vi "canDataSort.vi"() -> ()   [LabVIEW 2023] (continued)
      30\t75\tE0\t2E\t80\tFF\tFF\tFD\r\n      4322  0CF101A7   00000004    8        68\t00\t97\tCC\t00\t19\t39\tF2\r\n      4322  1FFFFFFF   00000004    8        00\t00\tFF\tFF\tFF\tFF\tFF\tFF\r\n      4312  1FFFFFFF   00000004    8        00\t20\tFF\tFF\tFF\tFF\tFF\tFF\r\n      4303  0CF102A7   00000004    8        30\t75\tE0\t2E\t80\tFF\tFF\tFD\r\n      4303  0CF101A7   00000004    8        68\t00\t97\tCC\t00\t19\t39\tF1\r\n      4302  1FFFFFFF   00000004    8        00\t00\tFF\tFF\tFF\tFF\tFF\tFF\r\n      4343  0C3C4D4A   00000004    8        BE\tFF\tFF\t7F\t18\tFF\tFF\t63\r\n      4343  0CF101A7   00000004    8        68\t00\t97\tCC\t00\t19\t39\tF3\r\n      4342  18F120F0   00000004    8        2B\t75\t60\tB1\tB0\t01\tFF\tFF\r\n      4341  18F11FF0   00000004    8        FF\t3F\t90\t68\t88\t1B\t10\t3C\r\n      4332  1FFFFFFF   00000004    8        00\t20\tFF\tFF\tFF\tFF\tFF\tFF\r\n      4323  0CF102A7   00000004    8        30\t75\tE0\t2E\t80\tFF\tFF\tFD\r\n      4322  0CF101A7   00000004    8        68\t00\t97\tCC\t00\t19\t39\tF2\r\n      4322  1FFFFFFF   00000004    8        00\t00\tFF\tFF\tFF\tFF\tFF\tFF\r\n      4312  1FFFFFFF   00000004    8        00\t20\tFF\tFF\tFF\tFF\tFF\tFF\r\n      4303  0CF102A7   00000004    8        30\t75\tE0\t2E\t80\tFF\tFF\tFD\r\n      4303  0CF101A7   00000004    8        68\t00\t97\tCC\t00\t19\t39\tF1\r\n      4344  0CF102A7   00000004    8        30\t75\tE0\t2E\t80\tFF\tFF\tFD\r\n      4343  0C3C4D4A   00000004    8        BE\tFF\tFF\t7F\t18\tFF\tFF\t63\r\n      4343  0CF101A7   00000004    8        68\t00\t97\tCC\t00\t19\t39\tF3\r\n      4342  18F120F0   00000004    8        2B\t75\t60\tB1\tB0\t01\tFF\tFF\r\n      4341  18F11FF0   00000004    8        FF\t3F\t90\t68\t88\t1B\t10\t3C\r\n      4332  1FFFFFFF   00000004    8        00\t20\tFF\tFF\tFF\tFF\tFF\tFF\r\n      4323  0CF102A7   00000004    8        30\t75\tE0\t2E\t80\tFF\tFF\tFD\r\n      4322  0CF101A7   00000004    8        68\t00\t97\tCC\t00\t19\t39\tF2\r\n      4322  1FFFFFFF   00000004    8        00\t00\tFF\tFF\tFF\tFF\tFF\tFF\r\n      4312  1FFFFFFF   00000004    8        00\t20\tFF\tFF\tFF\tFF\tFF\tFF\r\n      4303  0CF102A7   00000004    8        30\t75\tE0\t2E\t80\tFF\tFF\tFD\r\n      4344  0CF103A7   00000004    8        17\t1F\t08\t60\tB1\t1F\t08\t63\r\n      4344  0CF102A7   00000004    8        30\t75\tE0\t2E\t80\tFF\tFF\tFD\r\n      4343  0C3C4D4A   00000004    8        BE\tFF\tFF\t7F\t18\tFF\tFF\t63\r\n      4343  0CF101A7   00000004    8        68\t00\t97\tCC\t00\t19\t39\tF3\r\n      4342  18F120F0   00000004    8        2B\t75\t60\tB1\tB0\t01\tFF\tFF\r\n      4341  18F11FF0   00000004    8        FF\t3F\t90\t68\t88\t1B\t10\t3C\r\n      4332  1FFFFFFF   00000004    8        00\t20\tFF\tFF\tFF\tFF\tFF\tFF\r\n      4323  0CF102A7   00000004    8        30\t75\tE0\t2E\t80\tFF\tFF\tFD\r\n      4322  0CF101A7   00000004    8        68\t00\t97\tCC\t00\t19\t39\tF2\r\n      4322  1FFFFFFF   00000004    8        00\t00\tFF\tFF\tFF\tFF\tFF\tFF\r\n      4312  1FFFFFFF   00000004    8        00\t20\tFF\tFF\tFF\tFF\tFF\tFF\r\n      4345  0CF104A7   00000004    8        F0\t60\t22\tFC\tFF\tFF\tFF\t63\r\n      4344  0CF103A7   00000004    8        17\t1F\t08\t60\tB1\t1F\t08\t63\r\n      4344  0CF102A7   00000004    8        30\t75\tE0\t2E\t80\tFF\tFF\tFD\r\n      4343  0C3C4D4A   00000004    8        BE\tFF\tFF\t7F\t18\tFF\tFF\t63\r\n      4343  0CF101A7   00000004    8        68\t00\t97\tCC\t00\t19\t39\tF3\r\n      4342  18F120F0   00000004    8        2B\t75\t60\tB1\tB0\t01\tFF\tFF\r\n      4341  18F11FF0   00000004    8        FF\t3F\t90\t68\t88\t1B\t10\t3C\r\n      4332  1FFFFFFF   00000004    8        00\t20\tFF\tFF\tFF\tFF\tFF\tFF\r\n      4323  0CF102A7   00000004    8        30\t75\tE0\t2E\t80\tFF\tFF\tFD\r\n      4322  0CF101A7   00000004    8        68\t00\t97\tCC\t00\t19\t39\tF2\r\n      4322  1FFFFFFF   00000004    8        00\t00\tFF\tFF\tFF\tFF\tFF\tFF\r\n      4345  18F106A7   00000004    8        00\tF7\tFF\tFF\tFF\tFF\tFF\tC7\r\n      4345  0CF104A7   00000004    8        F0\t60\t22\tFC\tFF\tFF\tFF\t63\r\n      4344  0CF103A7   00000004    8        17\t1F\t08\t60\tB1\t1F\t08\t63\r\n      4344  0CF102A7   00000004    8        30\t75\tE0\t2E\t80\tFF\tFF\tFD\r\n      4343  0C3C4D4A   00000004    8        BE\tFF\tFF\t7F\t18\tFF\tFF\t63\r\n      4343  0CF101A7   00000004    8        68\t00\t97\tCC\t00\t19\t39\tF3\r\n      4342  18F120F0   00000004    8        2B\t75\t60\tB1\tB0\t01\tFF\tFF\r\n      4341  18F11FF0   00000004    8        FF\t3F\t90\t68\t88\t1B\t10\t3C\r\n      4332  1FFFFFFF   00000004    8        00\t20\tFF\tFF\tFF\tFF\tFF\tFF\r\n      4323  0CF102A7   00000004    8        30\t75\tE0\t2E\t80\tFF\tFF\tFD\r\n      4322  0CF101A7   00000004    8        68\t00\t97\tCC\t00\t19\t39\tF2\r\n      4346  18F121F0   00000004    8        09\t34\t00\t00\tFF\tFF\tB0\t01\r\n      4345  18F106A7   00000004    8        00\tF7\tFF\tFF\tFF\tFF\tFF\tC7\r\n      4345  0CF104A7   00000004    8        F0\t60\t22\tFC\tFF\tFF\tFF\t63\r\n      4344  0CF103A7   00000004    8        17\t1F\t08\t60\tB1\t1F\t08\t63\r\n      4344  0CF102A7   00000004    8        30\t75\tE0\t2E\t80\tFF\tFF\tFD\r\n      4343  0C3C4D4A   00000004    8        BE\tFF\tFF\t7F\t18\tFF\tFF\t63\r\n      4343  0CF101A7   00000004    8        68\t00\t97\tCC\t00\t19\t39\tF3\r\n      4342  18F120F0   00000004    8        2B\t75\t60\tB1\tB0\t01\tFF\tFF\r\n      4341  18F11FF0   00000004    8        FF\t3F\t90\t68\t88\t1B\t10\t3C\r\n      4332  1FFFFFFF   00000004    8        00\t20\tFF\tFF\tFF\tFF\tFF\tFF\r\n      4323  0CF102A7   00000004    8        30\t75\tE0\t2E\t80\tFF\tFF\tFD\r\n      4346  1FFFFFFF   00000004    8        00\t20\tFF\tFF\tFF\tFF\tFF\tFF\r\n      4346  18F121F0   00000004    8        09\t34\t00\t00\tFF\tFF\tB0\t01\r\n      4345  18F106A7   00000004    8        00\tF7\tFF\tFF\tFF\tFF\tFF\tC7\r\n      4345  0CF104A7   00000004    8        F0\t60\t22\tFC\tFF\tFF\tFF\t63\r\n      4344  0CF103A7   00000004    8        17\t1F\t08\t60\tB1\t1F\t08\t63\r\n      4344  0CF102A7   00000004    8        30\t75\tE0\t2E\t80\tFF\tFF\tFD\r\n      4343  0C3C4D4A   00000004    8        BE\tFF\tFF\t7F\t18\tFF\tFF\t63\r\n      4343  0CF101A7   00000004    8        68\t00\t97\tCC\t00\t19\t39\tF3\r\n      4342  18F120F0   00000004    8        2B\t75\t60\tB1\tB0\t01\tFF\tFF\r\n      4341  18F11FF0   00000004    8        FF\t3F\t90\t68\t88\t1B\t10\t3C\r\n      4332  1FFFFFFF   00000004    8        00\t20\tFF\tFF\tFF\tFF\tFF\tFF\r\n      4352  1FFFFFFF   00000004    8        00\t00\tFF\tFF\tFF\tFF\tFF\tFF\r\n      4346  1FFFFFFF   00000004    8        00\t20\tFF\tFF\tFF\tFF\tFF\tFF\r\n      4346  18F121F0   00000004    8        09\t34\t00\t00\tFF\tFF\tB0\t01\r\n      4345  18F106A7   00000004    8        00\tF7\tFF\tFF\tFF\tFF\tFF\tC7\r\n      4345  0CF104A7   00000004    8        F0\t60\t22\tFC\tFF\tFF\tFF\t63\r\n      4344  0CF103A7   00000004    8        17\t1F\t08\t60\tB1\t1F\t08\t63\r\n      4344  0CF102A7   00000004    8        30\t75\tE0\t2E\t80\tFF\tFF\tFD\r\n      4343  0C3C4D4A   00000004    8        BE\tFF\tFF\t7F\t18\tFF\tFF\t63\r\n      4343  0CF101A7   00000004    8        68\t00\t97\tCC\t00\t19\t39\tF3\r\n      4342  18F120F0   00000004    8        2B\t75\t60\tB1\tB0\t01\tFF\tFF\r\n      4341  18F11FF0   00000004    8        FF\t3F\t90\t68\t88\t1B\t10\t3C\r\n      4362  1FFFFFFF   00000004    8        00\t00\tFF\tFF\tFF\tFF\tFF\tFF\r\n      4352  1FFFFFFF   00000004    8        00\t00\tFF\tFF\tFF\tFF\tFF\tFF\r\n      4346  1FFFFFFF   00000004    8        00\t20\tFF\tFF\tFF\tFF\tFF\tFF\r\n      4346  18F121F0   00000004    8        09\t34\t00\t00\tFF\tFF\tB0\t01\r\n      4345  18F106A7   00000004    8        00\tF7\tFF\tFF\tFF\tFF\tFF\tC7\r\n      4345  0CF104A7   00000004    8        F0\t60\t22\tFC\tFF\tFF\tFF\t63\r\n      4344  0CF103A7   00000004    8        17\t1F\t08\t60\tB1\t1F\t08\t63\r\n      4344  0CF102A7   00000004    8        30\t75\tE0\t2E\t80\tFF\tFF\tFD\r\n      4343  0C3C4D4A   00000004    8        BE\tFF\tFF\t7F\t18\tFF\tFF\t63\r\n      4343  0CF101A7   00000004    8        68\t00\t97\tCC\t00\t19\t39\tF3\r\n      4342  18F120F0   00000004    8        2B\t75\t60\tB1\tB0\t01\tFF\tFF\r\n      4363  0CF101A7   00000004    8        68\t00\t97\tCC\t00\t19\t39\tF4\r\n      4362  1FFFFFFF   00000004    8        00\t00\tFF\tFF\tFF\tFF\tFF\tFF\r\n      4352  1FFFFFFF   00000004    8        00\t00\tFF\tFF\tFF\tFF\tFF\tFF\r\n      4346  1FFFFFFF   00000004    8        00\t20\tFF\tFF\tFF\tFF\tFF\tFF\r\n      4346  18F121F0   00000004    8        09\t34\t00\t00\tFF\tFF\tB0\t01\r\n      4345  18F106A7   00000004    8        00\tF7\tFF\tFF\tFF\tFF\tFF\tC7\r\n      4345  0CF104A7   00000004    8        F0\t60\t22\tFC\tFF\tFF\tFF\t63\r\n      4344  0CF103A7   00000004    8        17\t1F\t08\t60\tB1\t1F\t08\t63\r\n      4344  0CF102A7   00000004    8        30\t75\tE0\t2E\t80\tFF\tFF\tFD\r\n      4343  0C3C4D4A   00000004    8        BE\tFF\tFF\t7F\t18\tFF\tFF\t63\r\n      4343  0CF101A7   00000004    8        68\t00\t97\tCC\t00\t19\t39\tF3\r\n      4363  0CF102A7   00000004    8        30\t75\tE0\t2E\t80\tFF\tFF\tFD\r\n      4363  0CF101A7   00000004    8        68\t00\t97\tCC\t00\t19\t39\tF4\r\n      4362  1FFFFFFF   00000004    8        00\t00\tFF\tFF\tFF\tFF\tFF\tFF\r\n      4352  1FFFFFFF   00000004    8        00\t00\tFF\tFF\tFF\tFF\tFF\tFF\r\n      4346  1FFFFFFF   00000004    8        00\t20\tFF\tFF\tFF\tFF\tFF\tFF\r\n      4346  18F121F0   00000004    8        09\t34\t00\t00\tFF\tFF\tB0\t01\r\n      4345  18F106A7   00000004    8        00\tF7\tFF\tFF\tFF\tFF\tFF\tC7\r\n      4345  0CF104A7   00000004    8        F0\t60\t22\tFC\tFF\tFF\tFF\t63\r\n      4344  0CF103A7   00000004    8        17\t1F\t08\t60\tB1\t1F\t08\t63\r\n      4344  0CF102A7   00000004    8        30\t75\tE0\t2E\t80\tFF\tFF\tFD\r\n      4343  0C3C4D4A   00000004    8        BE\tFF\tFF\t7F\t18\tFF\tFF\t63\r\n      4372  1FFFFFFF   00000004    8        00\t00\tFF\tFF\tFF\tFF\tFF\tFF\r\n      4363  0CF102A7   00000004    8        30\t75\tE0\t2E\t80\tFF\tFF\tFD\r\n      4363  0CF101A7   00000004    8        68\t00\t97\tCC\t00\t19\t39\tF4\r\n      4362  1FFFFFFF   00000004    8        00\t00\tFF\tFF\tFF\tFF\tFF\tFF\r\n      4352  1FFFFFFF   00000004    8        00\t00\tFF\tFF\tFF\tFF\tFF\tFF\r\n      4346  1FFFFFFF   00000004    8        00\t20\tFF\tFF\tFF\tFF\tFF\tFF\r\n      4346  18F121F0   00000004    8        09\t34\t00\t00\tFF\tFF\tB0\t01\r\n      4345  18F106A7   00000004    8        00\tF7\tFF\tFF\tFF\tFF\tFF\tC7\r\n      4345  0CF104A7   00000004    8        F0\t60\t22\tFC\tFF\tFF\tFF\t63\r\n      4344  0CF103A7   00000004    8        17\t1F\t08\t60\tB1\t1F\t08\t63\r\n      4344  0CF102A7   00000004    8        30\t75\tE0\t2E\t80\tFF\tFF\tFD\r\n      4382  1FFFFFFF   00000004    8        00\t00\tFF\tFF\tFF\tFF\tFF\tFF\r\n      4372  1FFFFFFF   00000004    8        00\t00\tFF\tFF\tFF\tFF\tFF\tFF\r\n      4363  0CF102A7   00000004    8        30\t75\tE0\t2E\t80\tFF\tFF\tFD\r\n      4363  0CF101A7   00000004    8        68\t00\t97\tCC\t00\t19\t39\tF4\r\n      4362  1FFFFFFF   00000004    8        00\t00\tFF\tFF\tFF\tFF\tFF\tFF\r\n      4352  1FFFFFFF   00000004    8        00\t00\tFF\tFF\tFF\tFF\tFF\tFF\r\n      4346  1FFFFFFF   00000004    8        00\t20\tFF\tFF\tFF\tFF\tFF\tFF\r\n      4346  18F121F0   00000004    8        09\t34\t00\t00\tFF\tFF\tB0\t01\r\n      4345  18F106A7   00000004    8        00\tF7\tFF\tFF\tFF\tFF\tFF\tC7\r\n      4345  0CF104A7   00000004    8        F0\t60\t22\tFC\tFF\tFF\tFF\t63\r\n      4344  0CF103A7   00000004    8        17\t1F\t08\t60\tB1\t1F\t08\t63\r\n      4382  0CF101A7   00000004    8        68\t00\t97\tCC\t00\t19\t39\tF5\r\n      4382  1FFFFFFF   00000004    8        00\t00\tFF\tFF\tFF\tFF\tFF\tFF\r\n      4372  1FFFFFFF   00000004    8        00\t00\tFF\tFF\tFF\tFF\tFF\tFF\r\n      4363  0CF102A7   00000004    8        30\t75\tE0\t2E\t80\tFF\tFF\tFD\r\n      4363  0CF101A7   00000004    8        68\t00\t97\tCC\t00\t19\t39\tF4\r\n      4362  1FFFFFFF   00000004    8        00\t00\tFF\tFF\tFF\tFF\tFF\tFF\r\n      4352  1FFFFFFF   00000004    8        00\t00\tFF\tFF\tFF\tFF\tFF\tFF\r\n      4346  1FFFFFFF   00000004    8        00\t20\tFF\tFF\tFF\tFF\tFF\tFF\r\n      4346  18F121F0   00000004    8        09\t34\t00\t00\tFF\tFF\tB0\t01\r\n      4345  18F106A7   00000004    8        00\tF7\tFF\tFF\tFF\tFF\tFF\tC7\r\n      4345  0CF104A7   00000004    8        F0\t60\t22\tFC\tFF\tFF\tFF\t63\r\n      4383  0CF102A7   00000004    8        30\t75\tE0\t2E\t80\tFF\tFF\tFD\r\n      4382  0CF101A7   00000004    8        68\t00\t97\tCC\t00\t19\t39\tF5\r\n      4382  1FFFFFFF   00000004    8        00\t00\tFF\tFF\tFF\tFF\tFF\tFF\r\n      4372  1FFFFFFF   00000004    8        00\t00\tFF\tFF\tFF\tFF\tFF\tFF\r\n      4363  0CF102A7   00000004    8        30\t75\tE0\t2E\t80\tFF\tFF\tFD\r\n      4363  0CF101A7   00000004    8        68\t00\t97\tCC\t00\t19\t39\tF4\r\n      4362  1FFFFFFF   00000004    8        00\t00\tFF\tFF\tFF\tFF\tFF\tFF\r\n      4352  1FFFFFFF   00000004    8        00\t00\tFF\tFF\tFF\tFF\tFF\tFF\r\n      4346  1FFFFFFF   00000004    8        00\t20\tFF\tFF\tFF\tFF\tFF\tFF\r\n      4346  18F121F0   00000004    8        09\t34\t00\t00\tFF\tFF\tB0\t01\r\n      4345  18F106A7   00000004    8        00\tF7\tFF\tFF\tFF\tFF\tFF\tC7\r\n      4392  1FFFFFFF   00000004    8        00\t00\tFF\tFF\tFF\tFF\tFF\tFF\r\n      4383  0CF102A7   00000004    8        30\t75\tE0\t2E\t80\tFF\tFF\tFD\r\n      4382  0CF101A7   00000004    8        68\t00\t97\tCC\t00\t19\t39\tF5\r\n      4382  1FFFFFFF   00000004    8        00\t00\tFF\tFF\tFF\tFF\tFF\tFF\r\n      4372  1FFFFFFF   00000004    8        00\t00\tFF\tFF\tFF\tFF\tFF\tFF\r\n      4363  0CF102A7   00000004    8        30\t75\tE0\t2E\t80\tFF\tFF\tFD\r\n      4363  0CF101A7   00000004    8        68\t00\t97\tCC\t00\t19\t39\tF4\r\n      4362  1FFFFFFF   00000004    8        00\t00\tFF\tFF\tFF\tFF\tFF\tFF\r\n      4352  1FFFFFFF   00000004    8        00\t00\tFF\tFF\tFF\tFF\tFF\tFF\r\n      4346  1FFFFFFF   00000004    8        00\t20\tFF\tFF\tFF\tFF\tFF\tFF\r\n      4346  18F121F0   00000004    8        09\t34\t00\t00\tFF\tFF\tB0\t01\r\n      4393  18F106A7   00000004    8        00\tF7\tFF\tFF\tFF\tFF\tFF\tC8\r\n      4392  1FFFFFFF   00000004    8        00\t00\tFF\tFF\tFF\tFF\tFF\tFF\r\n      4383  0CF102A7   00000004    8        30\t75\tE0\t2E\t80\tFF\tFF\tFD\r\n      4382  0CF101A7   00000004    8        68\t00\t97\tCC\t00\t19\t39\tF5\r\n      4382  1FFFFFFF   00000004    8        00\t00\tFF\tFF\tFF\tFF\tFF\tFF\r\n      4372  1FFFFFFF   00000004    8        00\t00\tFF\tFF\tFF\tFF\tFF\tFF\r\n      4363  0CF102A7   00000004    8        30\t75\tE0\t2E\t80\tFF\tFF\tFD\r\n      4363  0CF101A7   00000004    8        68\t00\t97\tCC\t00\t19\t39\tF4\r\n      4362  1FFFFFFF   00000004    8        00\t00\tFF\tFF\tFF\tFF\tFF\tFF\r\n      4352  1FFFFFFF   00000004    8        00\t00\tFF\tFF\tFF\tFF\tFF\tFF\r\n      4346  1FFFFFFF   00000004    8        00\t20\tFF\tFF\tFF\tFF\tFF\tFF\r\n      4402  1FFFFFFF   00000004    8        00\t00\tFF\tFF\tFF\tFF\tFF\tFF\r\n      4393  18F106A7   00000004    8        00\tF7\tFF\tFF\tFF\tFF\tFF\tC8\r\n      4392  1FFFFFFF   00000004    8        00\t00\tFF\tFF\tFF\tFF\tFF\tFF\r\n      4383  0CF102A7   00000004    8        30\t75\tE0\t2E\t80\tFF\tFF\tFD\r\n      4382  0CF101A7   00000004    8        68\t00\t97\tCC\t00\t19\t39\tF5\r\n      4382  1FFFFFFF   00000004    8        00\t00\tFF\tFF\tFF\tFF\tFF\tFF\r\n      4372  1FFFFFFF   00000004    8        00\t00\tFF\tFF\tFF\tFF\tFF\tFF\r\n      4363  0CF102A7   00000004    8        30\t75\tE0\t2E\t80\tFF\tFF\tFD\r\n      4363  0CF101A7   00000004    8        68\t00\t97\tCC\t00\t19\t39\tF4\r\n      4362  1FFFFFFF   00000004    8        00\t00\tFF\tFF\tFF\tFF\tFF\tFF\r\n      4352  1FFFFFFF   00000004    8        00\t00\tFF\tFF\tFF\tFF\tFF\tFF\r\n      4403  0CF101A7   00000004    8        68\t00\t97\tCC\t00\t19\t39\tF6\r\n      4402  1FFFFFFF   00000004    8        00\t00\tFF\tFF\tFF\tFF\tFF\tFF\r\n      4393  18F106A7   00000004    8        00\tF7\tFF\tFF\tFF\tFF\tFF\tC8\r\n      4392  1FFFFFFF   00000004    8        00\t00\tFF\tFF\tFF\tFF\tFF\tFF\r\n      4383  0CF102A7   00000004    8        30\t75\tE0\t2E\t80\tFF\tFF\tFD\r\n      4382  0CF101A7   00000004    8        68\t00\t97\tCC\t00\t19\t39\tF5\r\n      4382  1FFFFFFF   00000004    8        00\t00\tFF\tFF\tFF\tFF\tFF\tFF\r\n      4372  1FFFFFFF   00000004    8        00\t00\tFF\tFF\tFF\tFF\tFF\tFF\r\n      4363  0CF102A7   00000004    8        30\t75\tE0\t2E\t80\tFF\tFF\tFD\r\n      4363  0CF101A7   00000004    8        68\t00\t97\tCC\t00\t19\t39\tF4\r\n      4362  1FFFFFFF   00000004    8        00\t00\tFF\tFF\tFF\tFF\tFF\tFF\r\n      4403  0CF102A7   00000004    8        30\t75\tE0\t2E\t80\tFF\tFF\tFD\r\n      4403  0CF101A7   00000004    8        68\t00\t97\tCC\t00\t19\t39\tF6\r\n      4402  1FFFFFFF   00000004    8        00\t00\tFF\tFF\tFF\tFF\tFF\tFF\r\n      4393  18F106A7   00000004    8        00\tF7\tFF\tFF\tFF\tFF\tFF\tC8\r\n      4392  1FFFFFFF   00000004    8        00\t00\tFF\tFF\tFF\tFF\tFF\tFF\r\n      4383  0CF102A7   00000004    8        30\t75\tE0\t2E\t80\tFF\tFF\tFD\r\n      4382  0CF101A7   00000004    8        68\t00\t97\tCC\t00\t19\t39\tF5\r\n      4382  1FFFFFFF   00000004    8        00\t00\tFF\tFF\tFF\tFF\tFF\tFF\r\n      4372  1FFFFFFF   00000004    8        00\t00\tFF\tFF\tFF\tFF\tFF\tFF\r\n      4363  0CF102A7   00000004    8        30\t75\tE0\t2E\t80\tFF\tFF\tFD\r\n      4363  0CF101A7   00000004    8        68\t00\t97\tCC\t00\t19\t39\tF4\r\n      4412  1FFFFFFF   00000004    8        00\t00\tFF\tFF\tFF\tFF\tFF\tFF\r\n      4403  0CF102A7   00000004    8        30\t75\tE0\t2E\t80\tFF\tFF\tFD\r\n      4403  0CF101A7   00000004    8        68\t00\t97\tCC\t00\t19\t39\tF6\r\n      4402  1FFFFFFF   00000004    8        00\t00\tFF\tFF\tFF\tFF\tFF\tFF\r\n      4393  18F106A7   00000004    8        00\tF7\tFF\tFF\tFF\tFF\tFF\tC8\r\n      4392  1FFFFFFF   00000004    8        00\t00\tFF\tFF\tFF\tFF\tFF\tFF\r\n      4383  0CF102A7   00000004    8        30\t75\tE0\t2E\t80\tFF\tFF\tFD\r\n      4382  0CF101A7   00000004    8        68\t00\t97\tCC\t00\t19\t39\tF5\r\n      4382  1FFFFFFF   00000004    8        00\t00\tFF\tFF\tFF\tFF\tFF\tFF\r\n      4372  1FFFFFFF   00000004    8        00\t00\tFF\tFF\tFF\tFF\tFF\tFF\r\n      4363  0CF102A7   00000004    8        30\t75\tE0\t2E\t80\tFF\tFF\tFD\r\n      4422  1FFFFFFF   00000004    8        00\t00\tFF\tFF\tFF\tFF\tFF\tFF\r\n      4412  1FFFFFFF   00000004    8        00\t00\tFF\tFF\tFF\tFF\tFF\tFF\r\n      4403  0CF102A7   00000004    8        30\t75\tE0\t2E\t80\tFF\tFF\tFD\r\n      4403  0CF101A7   00000004    8        68\t00\t97\tCC\t00\t19\t39\tF6\r\n      4402  1FFFFFFF   00000004    8        00\t00\tFF\tFF\tFF\tFF\tFF\tFF\r\n      4393  18F106A7   00000004    8        00\tF7\tFF\tFF\tFF\tFF\tFF\tC8\r\n      4392  1FFFFFFF   00000004    8        00\t00\tFF\tFF\tFF\tFF\tFF\tFF\r\n      4383  0CF102A7   00000004    8        30\t75\tE0\t2E\t80\tFF\tFF\tFD\r\n      4382  0CF101A7   00000004    8        68\t00\t97\tCC\t00\t19\t39\tF5\r\n      4382  1FFFFFFF   00000004    8        00\t00\tFF\tFF\tFF\tFF\tFF\tFF\r\n      4372  1FFFFFFF   00000004    8        00\t00\tFF\tFF\tFF\tFF\tFF\tFF\r\n      4423  0CF101A7   00000004    8        68\t00\t97\tCC\t00\t19\t39\tF7\r\n      4422  1FFFFFFF   00000004    8        00\t00\tFF\tFF\tFF\tFF\tFF\tFF\r\n      4412  1FFFFFFF   00000004    8        00\t00\tFF\tFF\tFF\tFF\tFF\tFF\r\n      4403  0CF102A7   00000004    8        30\t75\tE0\t2E\t80\tFF\tFF\tFD\r\n      4403  0CF101A7   00000004    8        68\t00\t97\tCC\t00\t19\t39\tF6\r\n      4402  1FFFFFFF   00000004    8        00\t00\tFF\tFF\tFF\tFF\tFF\tFF\r\n      4393  18F106A7   00000004    8        00\tF7\tFF\tFF\tFF\tFF\tFF\tC8\r\n      4392  1FFFFFFF   00000004    8        00\t00\tFF\tFF\tFF\tFF\tFF\tFF\r\n      4383  0CF102A7   00000004    8        30\t75\tE0\t2E\t80\tFF\tFF\tFD\r\n      4382  0CF101A7   00000004    8        68\t00\t97\tCC\t00\t19\t39\tF5\r\n      4382  1FFFFFFF   00000004    8        00\t00\tFF\tFF\tFF\tFF\tFF\tFF\r\n      4423  0CF102A7   00000004    8        30\t75\tE0\t2E\t80\tFF\tFF\tFD\r\n      4423  0CF101A7   00000004    8        68\t00\t97\tCC\t00\t19\t39\tF7\r\n      4422  1FFFFFFF   00000004    8        00\t00\tFF\tFF\tFF\tFF\tFF\tFF\r\n      4412  1FFFFFFF   00000004    8        00\t00\tFF\tFF\tFF\tFF\tFF\tFF\r\n      4403  0CF102A7   00000004    8        30\t75\tE0\t2E\t80\tFF\tFF\tFD\r\n      4403  0CF101A7   00000004    8        68\t00\t97\tCC\t00\t19\t39\tF6\r\n      4402  1FFFFFFF   00000004    8        00\t00\tFF\tFF\tFF\tFF\tFF\tFF\r\n      4393  18F106A7   00000004    8        00\tF7\tFF\tFF\tFF\tFF\tFF\tC8\r\n      4392  1FFFFFFF   00000004    8        00\t00\tFF\tFF\tFF\tFF\tFF\tFF\r\n      4383  0CF102A7   00000004    8        30\t75\tE0\t2E\t80\tFF\tFF\tFD\r\n      4382  0CF101A7   00000004    8        68\t00\t97\tCC\t00\t19\t39\tF5\r\n      4432  1FFFFFFF   00000004    8        00\t00\tFF\tFF\tFF\tFF\tFF\tFF\r\n      4423  0CF102A7   00000004    8        30\t75\tE0\t2E\t80\tFF\tFF\tFD\r\n      4423  0CF101A7   00000004    8        68\t00\t97\tCC\t00\t19\t39\tF7\r\n      4422  1FFFFFFF   00000004    8        00\t00\tFF\tFF\tFF\tFF\tFF\tFF\r\n      4412  1FFFFFFF   00000004    8        00\t00\tFF\tFF\tFF\tFF\tFF\tFF\r\n      4403  0CF102A7   00000004    8        30\t75\tE0\t2E\t80\tFF\tFF\tFD\r\n      4403  0CF101A7   00000004    8        68\t00\t97\tCC\t00\t19\t39\tF6\r\n      4402  1FFFFFFF   00000004    8        00\t00\tFF\tFF\tFF\tFF\tFF\tFF\r\n      4393  18F106A7   00000004    8        00\tF7\tFF\tFF\tFF\tFF\tFF\tC8\r\n      4392  1FFFFFFF   00000004    8        00\t00\tFF\tFF\tFF\tFF\tFF\tFF\r\n      4383  0CF102A7   00000004    8        30\t75\tE0\t2E\t80\tFF\tFF\tFD\r\n      4441  18F11FF0   00000004    8        FF\t3F\t90\t68\t88\t1B\t10\t4C\r\n      4432  1FFFFFFF   00000004    8        00\t00\tFF\tFF\tFF\tFF\tFF\tFF\r\n      4423  0CF102A7   00000004    8        30\t75\tE0\t2E\t80\tFF\tFF\tFD\r\n      4423  0CF101A7   00000004    8        68\t00\t97\tCC\t00\t19\t39\tF7\r\n      4422  1FFFFFFF   00000004    8        00\t00\tFF\tFF\tFF\tFF\tFF\tFF\r\n      4412  1FFFFFFF   00000004    8        00\t00\tFF\tFF\tFF\tFF\tFF\tFF\r\n      4403  0CF102A7   00000004    8        30\t75\tE0\t2E\t80\tFF\tFF\tFD\r\n      4403  0CF101A7   00000004    8        68\t00\t97\tCC\t00\t19\t39\tF6\r\n      4402  1FFFFFFF   00000004    8        00\t00\tFF\tFF\tFF\tFF\tFF\tFF\r\n      4393  18F106A7   00000004    8        00\tF7\tFF\tFF\tFF\tFF\tFF\tC8\r\n      4392  1FFFFFFF   00000004    8        00\t00\tFF\tFF\tFF\tFF\tFF\tFF\r\n      4442  18F120F0   00000004    8        2B\t75\t60\tB1\tB0\t01\tFF\tFF\r\n      4441  18F11FF0   00000004    8        FF\t3F\t90\t68\t88\t1B\t10\t4C\r\n      4432  1FFFFFFF   00000004    8        00\t00\tFF\tFF\tFF\tFF\tFF\tFF\r\n      4423  0CF102A7   00000004    8        30\t75\tE0\t2E\t80\tFF\tFF\tFD\r\n      4423  0CF101A7   00000004    8        68\t00\t97\tCC\t00\t19\t39\tF7\r\n      4422  1FFFFFFF   00000004    8        00\t00\tFF\tFF\tFF\tFF\tFF\tFF\r\n      4412  1FFFFFFF   00000004    8        00\t00\tFF\tFF\tFF\tFF\tFF\tFF\r\n      4403  0CF102A7   00000004    8        30\t75\tE0\t2E\t80\tFF\tFF\tFD\r\n      4403  0CF101A7   00000004    8        68\t00\t97\tCC\t00\t19\t39\tF6\r\n      4402  1FFFFFFF   00000004    8        00\t00\tFF\tFF\tFF\tFF\tFF\tFF\r\n      4393  18F106A7   00000004    8        00\tF7\tFF\tFF\tFF\tFF\tFF\tC8\r\n      4443  0CF101A7   00000004    8        68\t00\t97\tCC\t00\t19\t39\tF8\r\n      4442  18F120F0   00000004    8        2B\t75\t60\tB1\tB0\t01\tFF\tFF\r\n      4441  18F11FF0   00000004    8        FF\t3F\t90\t68\t88\t1B\t10\t4C\r\n      4432  1FFFFFFF   00000004    8        00\t00\tFF\tFF\tFF\tFF\tFF\tFF\r\n      4423  0CF102A7   00000004    8        30\t75\tE0\t2E\t80\tFF\tFF\tFD\r\n      4423  0CF101A7   00000004    8        68\t00\t97\tCC\t00\t19\t39\tF7\r\n      4422  1FFFFFFF   00000004    8        00\t00\tFF\tFF\tFF\tFF\tFF\tFF\r\n      4412  1FFFFFFF   00000004    8        00\t00\tFF\tFF\tFF\tFF\tFF\tFF\r\n      4403  0CF102A7   00000004    8        30\t75\tE0\t2E\t80\tFF\tFF\tFD\r\n      4403  0CF101A7   00000004    8        68\t00\t97\tCC\t00\t19\t39\tF6\r\n      4402  1FFFFFFF   00000004    8        00\t00\tFF\tFF\tFF\tFF\tFF\tFF\r\n      4443  0C3C4D4A   00000004    8        BE\tFF\tFF\t7F\t18\tFF\tFF\t64\r\n      4443  0CF101A7   00000004    8        68\t00\t97\tCC\t00\t19\t39\tF8\r\n      4442  18F120F0   00000004    8        2B\t75\t60\tB1\tB0\t01\tFF\tFF\r\n      4441  18F11FF0   00000004    8        FF\t3F\t90\t68\t88\t1B\t10\t4C\r\n      4432  1FFFFFFF   00000004    8        00\t00\tFF\tFF\tFF\tFF\tFF\tFF\r\n      4423  0CF102A7   00000004    8        30\t75\tE0\t2E\t80\tFF\tFF\tFD\r\n      4423  0CF101A7   00000004    8        68\t00\t97\tCC\t00\t19\t39\tF7\r\n      4422  1FFFFFFF   00000004    8        00\t00\tFF\tFF\tFF\tFF\tFF\tFF\r\n      4412  1FFFFFFF   00000004    8        00\t00\tFF\tFF\tFF\tFF\tFF\tFF\r\n      4403  0CF102A7   00000004    8        30\t75\tE0\t2E\t80\tFF\tFF\tFD\r\n      4403  0CF101A7   00000004    8        68\t00\t97\tCC\t00\t19\t39\tF6\r\n      4444  0CF102A7   00000004    8        30\t75\tE0\t2E\t80\tFF\tFF\tFD\r\n      4443  0C3C4D4A   00000004    8        BE\tFF\tFF\t7F\t18\tFF\tFF\t64\r\n      4443  0CF101A7   00000004    8        68\t00\t97\tCC\t00\t19\t39\tF8\r\n      4442  18F120F0   00000004    8        2B\t75\t60\tB1\tB0\t01\tFF\tFF\r\n      4441  18F11FF0   00000004    8        FF\t3F\t90\t68\t88\t1B\t10\t4C\r\n      4432  1FFFFFFF   00000004    8        00\t00\tFF\tFF\tFF\tFF\tFF\tFF\r\n      4423  0CF102A7   00000004    8        30\t75\tE0\t2E\t80\tFF\tFF\tFD\r\n      4423  0CF101A7   00000004    8        68\t00\t97\tCC\t00\t19\t39\tF7\r\n      4422  1FFFFFFF   00000004    8        00\t00\tFF\tFF\tFF\tFF\tFF\tFF\r\n      4412  1FFFFFFF   00000004    8        00\t00\tFF\tFF\tFF\tFF\tFF\tFF\r\n      4403  0CF102A7   00000004    8        30\t75\tE0\t2E\t80\tFF\tFF\tFD\r\n      4444  0CF103A7   00000004    8        17\t1F\t08\t60\tB1\t1F\t08\t64\r\n      4444  0CF102A7   00000004    8        30\t75\tE0\t2E\t80\tFF\tFF\tFD\r\n      4443  0C3C4D4A   00000004    8        BE\tFF\tFF\t7F\t18\tFF\tFF\t64\r\n      4443  0CF101A7   00000004    8        68\t00\t97\tCC\t00\t19\t39\tF8\r\n      4442  18F120F0   00000004    8        2B\t75\t60\tB1\tB0\t01\tFF\tFF\r\n      4441  18F11FF0   00000004    8        FF\t3F\t90\t68\t88\t1B\t10\t4C\r\n      4432  1FFFFFFF   00000004    8        00\t00\tFF\tFF\tFF\tFF\tFF\tFF\r\n      4423  0CF102A7   00000004    8        30\t75\tE0\t2E\t80\tFF\tFF\tFD\r\n      4423  0CF101A7   00000004    8        68\t00\t97\tCC\t00\t19\t39\tF7\r\n      4422  1FFFFFFF   00000004    8        00\t00\tFF\tFF\tFF\tFF\tFF\tFF\r\n      4412  1FFFFFFF   00000004    8        00\t00\tFF\tFF\tFF\tFF\tFF\tFF\r\n      4445  0CF104A7   00000004    8        F0\t60\t22\tFC\tFF\tFF\tFF\t64\r\n      4444  0CF103A7   00000004    8        17\t1F\t08\t60\tB1\t1F\t08\t64\r\n      4444  0CF102A7   00000004    8        30\t75\tE0\t2E\t80\tFF\tFF\tFD\r\n      4443  0C3C4D4A   00000004    8        BE\tFF\tFF\t7F\t18\tFF\tFF\t64\r\n      4443  0CF101A7   00000004    8        68\t00\t97\tCC\t00\t19\t39\tF8\r\n      4442  18F120F0   00000004    8        2B\t75\t60\tB1\tB0\t01\tFF\tFF\r\n      4441  18F11FF0   00000004    8        FF\t3F\t90\t68\t88\t1B\t10\t4C\r\n      4432  1FFFFFFF   00000004    8        00\t00\tFF\tFF\tFF\tFF\tFF\tFF\r\n      4423  0CF102A7   00000004    8        30\t75\tE0\t2E\t80\tFF\tFF\tFD\r\n      4423  0CF101A7   00000004    8        68\t00\t97\tCC\t00\t19\t39\tF7\r\n      4422  1FFFFFFF   00000004    8        00\t00\tFF\tFF\tFF\tFF\tFF\tFF\r\n      4445  18F106A7   00000004    8        00\tF7\tFF\tFF\tFF\tFF\tFF\tC9\r\n      4445  0CF104A7   00000004    8        F0\t60\t22\tFC\tFF\tFF\tFF\t64\r\n      4444  0CF103A7   00000004    8        17\t1F\t08\t60\tB1\t1F\t08\t64\r\n      4444  0CF102A7   00000004    8        30\t75\tE0\t2E\t80\tFF\tFF\tFD\r\n      4443  0C3C4D4A   00000004    8        BE\tFF\tFF\t7F\t18\tFF\tFF\t64\r\n      4443  0CF101A7   00000004    8        68\t00\t97\tCC\t00\t19\t39\tF8\r\n      4442  18F120F0   00000004    8        2B\t75\t60\tB1\tB0\t01\tFF\tFF\r\n      4441  18F11FF0   00000004    8        FF\t3F\t90\t68\t88\t1B\t10\t4C\r\n      4432  1FFFFFFF   00000004    8        00\t00\tFF\tFF\tFF\tFF\tFF\tFF\r\n      4423  0CF102A7   00000004    8        30\t75\tE0\t2E\t80\tFF\tFF\tFD\r\n      4423  0CF101A7   00000004    8        68\t00\t97\tCC\t00\t19\t39\tF7\r\n      4446  18F121F0   00000004    8        09\t34\t00\t00\tFF\tFF\tB0\t01\r\n      4445  18F106A7   00000004    8        00\tF7\tFF\tFF\tFF\tFF\tFF\tC9\r\n      4445  0CF104A7   00000004    8        F0\t60\t22\tFC\tFF\tFF\tFF\t64\r\n      4444  0CF103A7   00000004    8        17\t1F\t08\t60\tB1\t1F\t08\t64\r\n      4444  0CF102A7   00000004    8        30\t75\tE0\t2E\t80\tFF\tFF\tFD\r\n      4443  0C3C4D4A   00000004    8        BE\tFF\tFF\t7F\t18\tFF\tFF\t64\r\n      4443  0CF101A7   00000004    8        68\t00\t97\tCC\t00\t19\t39\tF8\r\n      4442  18F120F0   00000004    8        2B\t75\t60\tB1\tB0\t01\tFF\tFF\r\n      4441  18F11FF0   00000004    8        FF\t3F\t90\t68\t88\t1B\t10\t4C\r\n      4432  1FFFFFFF   00000004    8        00\t00\tFF\tFF\tFF\tFF\tFF\tFF\r\n      4423  0CF102A7   00000004    8        30\t75\tE0\t2E\t80\tFF\tFF\tFD\r\n      4446  1FFFFFFF   00000004    8        00\t00\tFF\tFF\tFF\tFF\tFF\tFF\r\n      4446  18F121F0   00000004    8        09\t34\t00\t00\tFF\tFF\tB0\t01\r\n      4445  18F106A7   00000004    8        00\tF7\tFF\tFF\tFF\tFF\tFF\tC9\r\n      4445  0CF104A7   00000004    8        F0\t60\t22\tFC\tFF\tFF\tFF\t64\r\n      4444  0CF103A7   00000004    8        17\t1F\t08\t60\tB1\t1F\t08\t64\r\n      4444  0CF102A7   00000004    8        30\t75\tE0\t2E\t80\tFF\tFF\tFD\r\n      4443  0C3C4D4A   00000004    8        BE\tFF\tFF\t7F\t18\tFF\tFF\t64\r\n      4443  0CF101A7   00000004    8        68\t00\t97\tCC\t00\t19\t39\tF8\r\n      4442  18F120F0   00000004    8        2B\t75\t60\tB1\tB0\t01\tFF\tFF\r\n      4441  18F11FF0   00000004    8        FF\t3F\t90\t68\t88\t1B\t10\t4C\r\n      4432  1FFFFFFF   00000004    8        00\t00\tFF\tFF\tFF\tFF\tFF\tFF\r\n      4452  1FFFFFFF   00000004    8        00\t00\tFF\tFF\tFF\tFF\tFF\tFF\r\n      4446  1FFFFFFF   00000004    8        00\t00\tFF\tFF\tFF\tFF\tFF\tFF\r\n      4446  18F121F0   00000004    8        09\t34\t00\t00\tFF\tFF\tB0\t01\r\n      4445  18F106A7   00000004    8        00\tF7\tFF\tFF\tFF\tFF\tFF\tC9\r\n      4445  0CF104A7   00000004    8        F0\t60\t22\tFC\tFF\tFF\tFF\t64\r\n      4444  0CF103A7   00000004    8        17\t1F\t08\t60\tB1\t1F\t08\t64\r\n      4444  0CF102A7   00000004    8        30\t75\tE0\t2E\t80\tFF\tFF\tFD\r\n      4443  0C3C4D4A   00000004    8        BE\tFF\tFF\t7F\t18\tFF\tFF\t64\r\n      4443  0CF101A7   00000004    8        68\t00\t97\tCC\t00\t19\t39\tF8\r\n      4442  18F120F0   00000004    8        2B\t75\t60\tB1\tB0\t01\tFF\tFF\r\n      4441  18F11FF0   00000004    8        FF\t3F\t90\t68\t88\t1B\t10\t4C\r\n      4462  1FFFFFFF   00000004    8        00\t00\tFF\tFF\tFF\tFF\tFF\tFF\r\n      4452  1FFFFFFF   00000004    8        00\t00\tFF\tFF\tFF\tFF\tFF\tFF\r\n      4446  1FFFFFFF   00000004    8        00\t00\tFF\tFF\tFF\tFF\tFF\tFF\r\n      4446  18F121F0   00000004    8        09\t34\t00\t00\tFF\tFF\tB0\t01\r\n      4445  18F106A7   00000004    8        00\tF7\tFF\tFF\tFF\tFF\tFF\tC9\r\n      4445  0CF104A7   00000004    8        F0\t60\t22\tFC\tFF\tFF\tFF\t64\r\n      4444  0CF103A7   00000004    8        17\t1F\t08\t60\tB1\t1F\t08\t64\r\n      4444  0CF102A7   00000004    8        30\t75\tE0\t2E\t80\tFF\tFF\tFD\r\n      4443  0C3C4D4A   00000004    8        BE\tFF\tFF\t7F\t18\tFF\tFF\t64\r\n      4443  0CF101A7   00000004    8        68\t00\t97\tCC\t00\t19\t39\tF8\r\n      4442  18F120F0   00000004    8        2B\t75\t60\tB1\tB0\t01\tFF\tFF\r\n      4463  0CF101A7   00000004    8        68\t00\t97\tCC\t00\t19\t39\tF9\r\n      4462  1FFFFFFF   00000004    8        00\t00\tFF\tFF\tFF\tFF\tFF\tFF\r\n      4452  1FFFFFFF   00000004    8        00\t00\tFF\tFF\tFF\tFF\tFF\tFF\r\n      4446  1FFFFFFF   00000004    8        00\t00\tFF\tFF\tFF\tFF\tFF\tFF\r\n      4446  18F121F0   00000004    8        09\t34\t00\t00\tFF\tFF\tB0\t01\r\n      4445  18F106A7   00000004    8        00\tF7\tFF\tFF\tFF\tFF\tFF\tC9\r\n      4445  0CF104A7   00000004    8        F0\t60\t22\tFC\tFF\tFF\tFF\t64\r\n      4444  0CF103A7   00000004    8        17\t1F\t08\t60\tB1\t1F\t08\t64\r\n      4444  0CF102A7   00000004    8        30\t75\tE0\t2E\t80\tFF\tFF\tFD\r\n      4443  0C3C4D4A   00000004    8        BE\tFF\tFF\t7F\t18\tFF\tFF\t64\r\n      4443  0CF101A7   00000004    8        68\t00\t97\tCC\t00\t19\t39\tF8\r\n      4463  0CF102A7   00000004    8        30\t75\tE0\t2E\t80\tFF\tFF\tFD\r\n      4463  0CF101A7   00000004    8        68\t00\t97\tCC\t00\t19\t39\tF9\r\n      4462  1FFFFFFF   00000004    8        00\t00\tFF\tFF\tFF\tFF\tFF\tFF\r\n      4452  1FFFFFFF   00000004    8        00\t00\tFF\tFF\tFF\tFF\tFF\tFF\r\n      4446  1FFFFFFF   00000004    8        00\t00\tFF\tFF\tFF\tFF\tFF\tFF\r\n      4446  18F121F0   00000004    8        09\t34\t00\t00\tFF\tFF\tB0\t01\r\n      4445  18F106A7   00000004    8        00\tF7\tFF\tFF\tFF\tFF\tFF\tC9\r\n      4445  0CF104A7   00000004    8        F0\t60\t22\tFC\tFF\tFF\tFF\t64\r\n      4444  0CF103A7   00000004    8        17\t1F\t08\t60\tB1\t1F\t08\t64\r\n      4444  0CF102A7   00000004    8        30\t75\tE0\t2E\t80\tFF\tFF\tFD\r\n      4443  0C3C4D4A   00000004    8        BE\tFF\tFF\t7F\t18\tFF\tFF\t64\r\n      4472  1FFFFFFF   00000004    8        00\t00\tFF\tFF\tFF\tFF\tFF\tFF\r\n      4463  0CF102A7   00000004    8        30\t75\tE0\t2E\t80\tFF\tFF\tFD\r\n      4463  0CF101A7   00000004    8        68\t00\t97\tCC\t00\t19\t39\tF9\r\n      4462  1FFFFFFF   00000004    8        00\t00\tFF\tFF\tFF\tFF\tFF\tFF\r\n      4452  1FFFFFFF   00000004    8        00\t00\tFF\tFF\tFF\tFF\tFF\tFF\r\n      4446  1FFFFFFF   00000004    8        00\t00\tFF\tFF\tFF\tFF\tFF\tFF\r\n      4446  18F121F0   00000004    8        09\t34\t00\t00\tFF\tFF\tB0\t01\r\n      4445  18F106A7   00000004    8        00\tF7\tFF\tFF\tFF\tFF\tFF\tC9\r\n      4445  0CF104A7   00000004    8        F0\t60\t22\tFC\tFF\tFF\tFF\t64\r\n      4444  0CF103A7   00000004    8        17\t1F\t08\t60\tB1\t1F\t08\t64\r\n      4444  0CF102A7   00000004    8        30\t75\tE0\t2E\t80\tFF\tFF\tFD\r\n      4482  1FFFFFFF   00000004    8        00\t00\tFF\tFF\tFF\tFF\tFF\tFF\r\n      4472  1FFFFFFF   00000004    8        00\t00\tFF\tFF\tFF\tFF\tFF\tFF\r\n      4463  0CF102A7   00000004    8        30\t75\tE0\t2E\t80\tFF\tFF\tFD\r\n      4463  0CF101A7   00000004    8        68\t00\t97\tCC\t00\t19\t39\tF9\r\n      4462  1FFFFFFF   00000004    8        00\t00\tFF\tFF\tFF\tFF\tFF\tFF\r\n      4452  1FFFFFFF   00000004    8        00\t00\tFF\tFF\tFF\tFF\tFF\tFF\r\n      4446  1FFFFFFF   00000004    8        00\t00\tFF\tFF\tFF\tFF\tFF\tFF\r\n      4446  18F121F0   00000004    8        09\t34\t00\t00\tFF\tFF\tB0\t01\r\n      4445  18F106A7   00000004    8        00\tF7\tFF\tFF\tFF\tFF\tFF\tC9\r\n      4445  0CF104A7   00000004    8        F0\t60\t22\tFC\tFF\tFF\tFF\t64\r\n      4444  0CF103A7   00000004    8        17\t1F\t08\t60\tB1\t1F\t08\t64\r\n      4482  0CF101A7   00000004    8        68\t00\t97\tCC\t00\t19\t39\tFA\r\n      4482  1FFFFFFF   00000004    8        00\t00\tFF\tFF\tFF\tFF\tFF\tFF\r\n      4472  1FFFFFFF   00000004    8        00\t00\tFF\tFF\tFF\tFF\tFF\tFF\r\n      4463  0CF102A7   00000004    8        30\t75\tE0\t2E\t80\tFF\tFF\tFD\r\n      4463  0CF101A7   00000004    8        68\t00\t97\tCC\t00\t19\t39\tF9\r\n      4462  1FFFFFFF   00000004    8        00\t00\tFF\tFF\tFF\tFF\tFF\tFF\r\n      4452  1FFFFFFF   00000004    8        00\t00\tFF\tFF\tFF\tFF\tFF\tFF\r\n      4446  1FFFFFFF   00000004    8        00\t00\tFF\tFF\tFF\tFF\tFF\tFF\r\n      4446  18F121F0   00000004    8        09\t34\t00\t00\tFF\tFF\tB0\t01\r\n      4445  18F106A7   00000004    8        00\tF7\tFF\tFF\tFF\tFF\tFF\tC9\r\n      4445  0CF104A7   00000004    8        F0\t60\t22\tFC\tFF\tFF\tFF\t64\r\n      4483  0CF102A7   00000004    8        30\t75\tE0\t2E\t80\tFF\tFF\tFD\r\n      4482  0CF101A7   00000004    8        68\t00\t97\tCC\t00\t19\t39\tFA\r\n      4482  1FFFFFFF   00000004    8        00\t00\tFF\tFF\tFF\tFF\tFF\tFF\r\n      4472  1FFFFFFF   00000004    8        00\t00\tFF\tFF\tFF\tFF\tFF\tFF\r\n      4463  0CF102A7   00000004    8        30\t75\tE0\t2E\t80\tFF\tFF\tFD\r\n      4463  0CF101A7   00000004    8        68\t00\t97\tCC\t00\t19\t39\tF9\r\n      4462  1FFFFFFF   00000004    8        00\t00\tFF\tFF\tFF\tFF\tFF\tFF\r\n      4452  1FFFFFFF   00000004    8        00\t00\tFF\tFF\tFF\tFF\tFF\tFF\r\n      4446  1FFFFFFF   00000004    8        00\t00\tFF\tFF\tFF\tFF\tFF\tFF\r\n      4446  18F121F0   00000004    8        09\t34\t00\t00\tFF\tFF\tB0\t01\r\n      4445  18F106A7   00000004    8        00\tF7\tFF\tFF\tFF\tFF\tFF\tC9\r\n      4492  1FFFFFFF   00000004    8        00\t20\tFF\tFF\tFF\tFF\tFF\tFF\r\n      4483  0CF102A7   00000004    8        30\t75\tE0\t2E\t80\tFF\tFF\tFD\r\n      4482  0CF101A7   00000004    8        68\t00\t97\tCC\t00\t19\t39\tFA\r\n      4482  1FFFFFFF   00000004    8        00\t00\tFF\tFF\tFF\tFF\tFF\tFF\r\n      4472  1FFFFFFF   00000004    8        00\t00\tFF\tFF\tFF\tFF\tFF\tFF\r\n      4463  0CF102A7   00000004    8        30\t75\tE0\t2E\t80\tFF\tFF\tFD\r\n      4463  0CF101A7   00000004    8        68\t00\t97\tCC\t00\t19\t39\tF9\r\n      4462  1FFFFFFF   00000004    8        00\t00\tFF\tFF\tFF\tFF\tFF\tFF\r\n      4452  1FFFFFFF   00000004    8        00\t00\tFF\tFF\tFF\tFF\tFF\tFF\r\n      4446  1FFFFFFF   00000004    8        00\t00\tFF\tFF\tFF\tFF\tFF\tFF\r\n      4446  18F121F0   00000004    8        09\t34\t00\t00\tFF\tFF\tB0\t01\r\n      4493  18F106A7   00000004    8        00\tF7\tFF\tFF\tFF\tFF\tFF\tCA\r\n      4492  1FFFFFFF   00000004    8        00\t20\tFF\tFF\tFF\tFF\tFF\tFF\r\n      4483  0CF102A7   00000004    8        30\t75\tE0\t2E\t80\tFF\tFF\tFD\r\n      4482  0CF101A7   00000004    8        68\t00\t97\tCC\t00\t19\t39\tFA\r\n      4482  1FFFFFFF   00000004    8        00\t00\tFF\tFF\tFF\tFF\tFF\tFF\r\n      4472  1FFFFFFF   00000004    8        00\t00\tFF\tFF\tFF\tFF\tFF\tFF\r\n      4463  0CF102A7   00000004    8        30\t75\tE0\t2E\t80\tFF\tFF\tFD\r\n      4463  0CF101A7   00000004    8        68\t00\t97\tCC\t00\t19\t39\tF9\r\n      4462  1FFFFFFF   00000004    8        00\t00\tFF\tFF\tFF\tFF\tFF\tFF\r\n      4452  1FFFFFFF   00000004    8        00\t00\tFF\tFF\tFF\tFF\tFF\tFF\r\n      4446  1FFFFFFF   00000004    8        00\t00\tFF\tFF\tFF\tFF\tFF\tFF\r\n      4502  1FFFFFFF   00000004    8        00\t00\tFF\tFF\tFF\tFF\tFF\tFF\r\n      4493  18F106A7   00000004    8        00\tF7\tFF\tFF\tFF\tFF\tFF\tCA\r\n      4492  1FFFFFFF   00000004    8        00\t20\tFF\tFF\tFF\tFF\tFF\tFF\r\n      4483  0CF102A7   00000004    8        30\t75\tE0\t2E\t80\tFF\tFF\tFD\r\n      4482  0CF101A7   00000004    8        68\t00\t97\tCC\t00\t19\t39\tFA\r\n      4482  1FFFFFFF   00000004    8        00\t00\tFF\tFF\tFF\tFF\tFF\tFF\r\n      4472  1FFFFFFF   00000004    8        00\t00\tFF\tFF\tFF\tFF\tFF\tFF\r\n      4463  0CF102A7   00000004    8        30\t75\tE0\t2E\t80\tFF\tFF\tFD\r\n      4463  0CF101A7   00000004    8        68\t00\t97\tCC\t00\t19\t39\tF9\r\n      4462  1FFFFFFF   00000004    8        00\t00\tFF\tFF\tFF\tFF\tFF\tFF\r\n      4452  1FFFFFFF   00000004    8        00\t00\tFF\tFF\tFF\tFF\tFF\tFF\r\n      4503  0CF101A7   00000004    
